vi "STM Read Meta Data (UDP Ref).vi"(6 "Options":T4={"Ignore Timeout Error"=TRUE, "timeout ms (1000)"=1000, "max size (548)"=548}, 8 "error in":errorcluster, 11 "connection ID":refnum<k16>) -> (0 "error out":errorcluster, 1 "Meta data":T1[](array[typedef]), 3 "Connection Info Out":T2, 4 "data info":T3)   [LabVIEW 2013]
doc: "This VI reads the meta data information from a remote computer. Use this VI to retrieve the variable names and types that a remote computer exports.\n\nThis VI parses the data and returns a cluster containing the meta data information."
uses:
  stm_UDP Read Options.ctl
  stm_UDP Data Info.ctl
  stm_UDP Connection Info.ctl
  stm_MetaDataElement.ctl
  UDP/Read Meta Data (UDP Clst).vi
  NI STM.lvlib
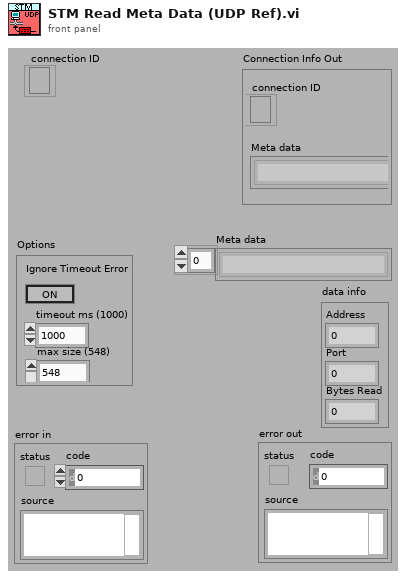
[diagram p1: front panel]
types:
  T1 = typedef "stm_MetaDataElement.ctl" = string
  T2 = typedef "stm_UDP Connection Info.ctl" = cluster{"connection ID":refnum<k16>, "Meta data":T1[]}
  T3 = typedef "stm_UDP Data Info.ctl" = cluster{"Address":u32, "Port":u16, "Bytes Read":i32}
  T4 = typedef "stm_UDP Read Options.ctl" = cluster{"Ignore Timeout Error":bool, "timeout ms (1000)":i32, "max size (548)":i32}
  T5 = typedef "NI STM.lvlib/MetaDataElement.ctl" = string
  T6 = typedef "NI STM.lvlib/UDP Connection Info.ctl" = cluster{"connection ID":refnum<k16>, "meta data":T5[]}
  T7 = typedef "NI STM.lvlib/UDP Data Info.ctl" = cluster{"address":u32, "port":u16, "bytes read":i32}
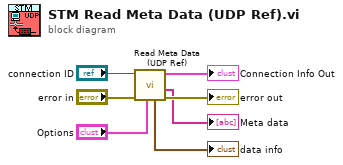
[diagram p0: block diagram]
diagram:
  n1 = call "Read Meta Data (UDP Ref).vi"("options"="Options", "error in"="error in", "connection ID"="connection ID") -> ("error out"=→"error out":errorcluster, "meta data"=→"Meta data":T5[], "connection info out"=→"Connection Info Out":T6, "data info"=→"data info":T7)  [unwired: 5 in]
